vi "Accelerometer_LPF.vi"() -> ()   [LabVIEW 2025]
uses:
  <vilib>/Analysis/NI_AALBase.lvlib
panel:
  in  "Lambda":dbl=0.7 min=0.0 max=1.0
  out "Low Pass Filter":dbl[][](graph)
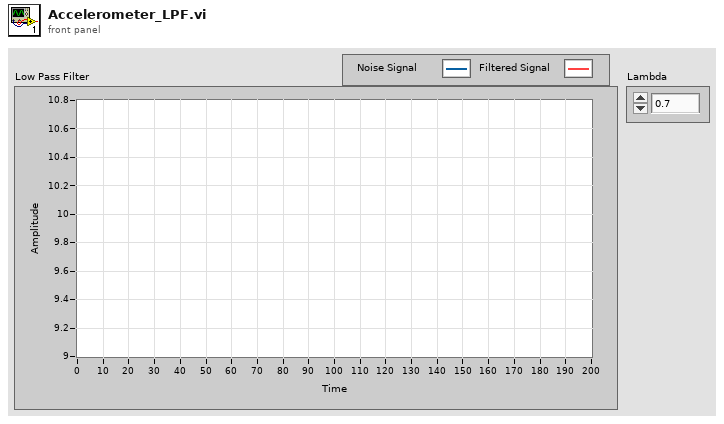
[diagram p1: front panel]
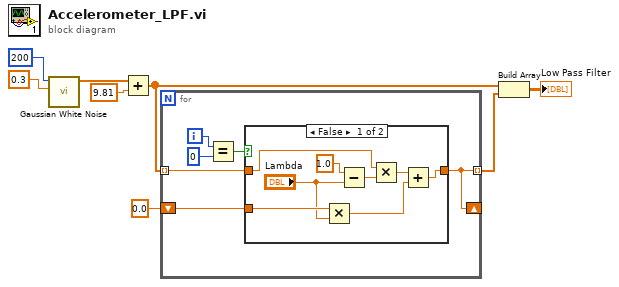
[diagram p0: block diagram]
diagram:
  n1 = call <vilib>:"Gaussian White Noise.vi"("standard deviation"=0.3, "samples"=200) -> ("Gaussian noise pattern"=w6:dbl[])  [unwired: 8 in, 1 out]
  n2 = Add(x=w6, y=9.81) -> (x+y=w3:dbl[])
  n3 = for {
    tunnel: w3 -> [w11] mode=indexing
    tunnel: [w10] -> w2 mode=indexing
    shift-right: [w10] -> _
    shift-left: 0.0 -> [w9]
    i -> [w13]
    n4 = Equal?(x=w13, y=0) -> (x = y?=w14:bool)
    n5 = case shown="False" w14 {
      tunnel: w11 -> [w20 w23]
      tunnel: [w15 w23] -> w10
      tunnel: w9 -> [w22 _]
      frame False {
        n6 = Multiply(x=w22, y="Lambda") -> (x*y=w21:dbl)
        n7 = Subtract(x=1.0, y="Lambda") -> (x-y=w19:dbl)
        n8 = Multiply(x=w20, y=w19) -> (x*y=w16:dbl)
        n9 = Add(x=w16, y=w21) -> (x+y=w15:dbl)
      }
      frame True {
      }
    }
  }
  n10 = Build Array(w3, w2) -> (→"Low Pass Filter":dbl[][])
